vi "Close.vi"(8 "error in (no error)":errorcluster, 11 "TCP Stream in":refnum<class "TCP Stream.lvclass">) -> (0 "error out":errorcluster, 3 "TCP Stream out":refnum<class "TCP Stream.lvclass">)   [LabVIEW 2020, in "Stream-TCP.lvlib" / "TCP Stream.lvclass"]
uses:
  TCP Stream.lvclass
  lv-stream/stream/Stream/Stream.lvclass
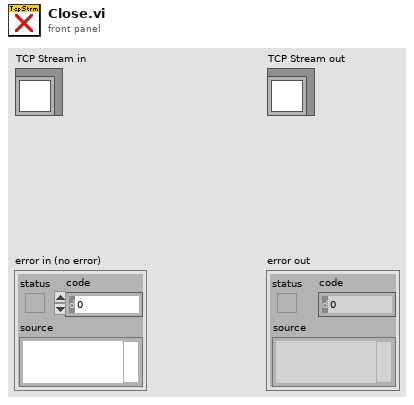
[diagram p1: front panel]
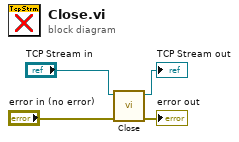
[diagram p0: block diagram]
diagram:
  n1 = call-parent "Close.vi"("error in (no error)"="error in (no error)", "Stream in"="TCP Stream in") -> ("error out"=→"error out":errorcluster, "Stream out"=→"TCP Stream out":refnum<class "TCP Stream.lvclass">)  [unwired: 8 in]
